vi "OverrideHandler.vi"() -> ()   [LabVIEW 2011]
uses:
  SailBot/ProgrammingRepo/Software/2-RIO/2 Typedefs/setpoints to boat.ctl
  SailBot/ProgrammingRepo/Software/2-RIO/2 Typedefs/sail setpt.ctl
  SailBot/ProgrammingRepo/Software/2-RIO/2 Typedefs/rudder angle.ctl
  SailBot/ProgrammingRepo/Software/2-RIO/2 Globals/2 Global.vi
panel:
  out "Think Setpoints":cluster{"Rudder Angle":T1, "Sail Position":T2}
  out "Override Active":bool
  out "Override Setpoints":T3
  in  "VI Stop":bool
  out "Setpoints to Boat":T3
  # "This is the Override Handler: \nIt checks to see if the manual override has been activated, and sends setpoints to the boat based on that boolean.\n\nTODO: Check to make sure that rudder and sail are always communicated as (0) = rudder and (1) = sail."
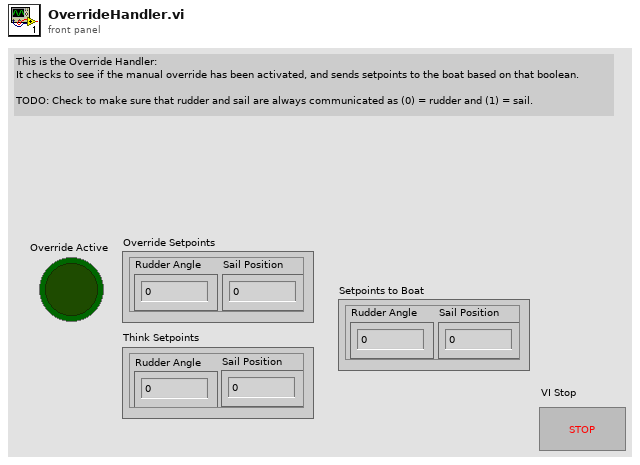
[diagram p1: front panel]
types:
  T1 = typedef "rudder angle.ctl" = dbl
  T2 = typedef "sail setpt.ctl" = dbl
  T3 = typedef "setpoints to boat.ctl" = cluster{"Sail Position":T2, "Rudder Angle":T1}
  T4 = typedef "manual override.ctl" = cluster{"Override Active":bool, "Setpoints":T3}
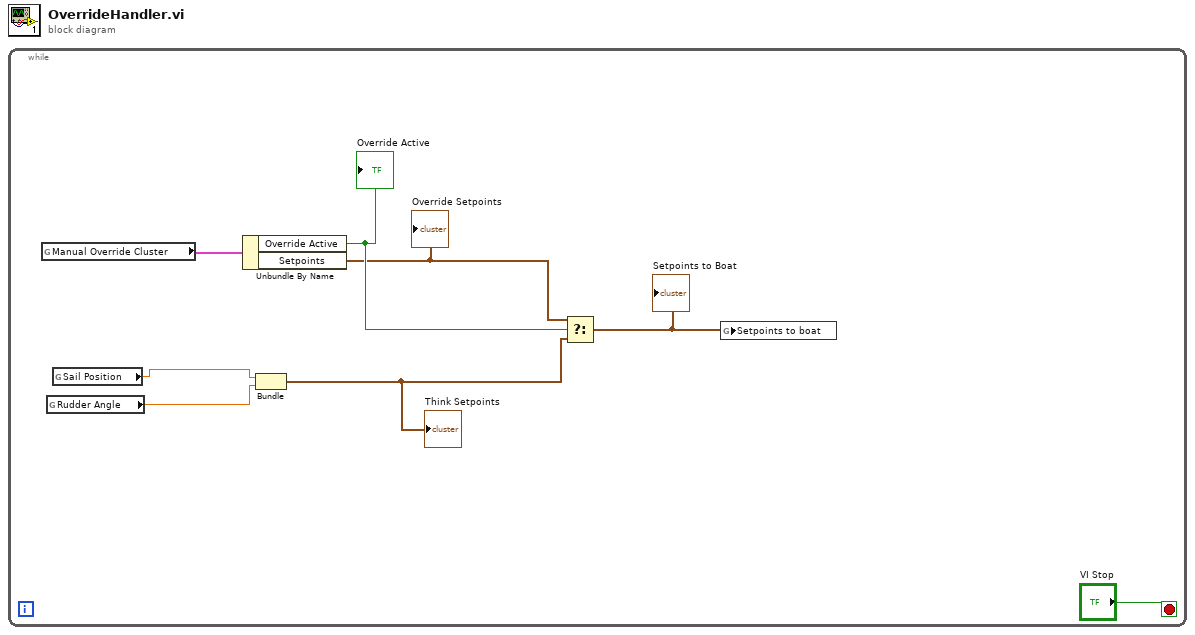
[diagram p0: block diagram]
diagram:
  n1 = while {
    stop <- "VI Stop" stop-if-true
    n2 = global read "2 Global.vi" "Manual Override Cluster"() -> (w8:T4)
    n3 = global read "2 Global.vi" "Rudder Angle"() -> (w4:T1)
    n4 = global read "2 Global.vi" "Sail Position"() -> (w5:T2)
    n5 = Unbundle By Name(w8) -> ("Override Active"=w7:bool, "Setpoints"=w6:T3)
    "Override Setpoints" <- w6
    "Override Active" <- w7
    n6 = Bundle("Sail Position"=w5, "Rudder Angle"=w4) -> (w1:cluster{"Sail Position":T2, "Rudder Angle":T1})  [unwired: 1 in]
    "Think Setpoints" <- w1
    n7 = Select(t=w6, s=w7, f=w1) -> (s? t:f=w3:T3)
    "Setpoints to Boat" <- w3
    n8 = global write "2 Global.vi" "Setpoints to boat"(w3) -> ()
  }
